vi "reference_cluster.vi"(0 "control cluster":T5, 3 "error in":errorcluster) -> (4 "error event refnum":refnum<event-registration>, 5 "reference cluster":T6, 8 "error out":errorcluster)   [LabVIEW 2016]
uses:
  Type Definitions/reference_cluster.ctl
  Type Definitions/vars_settings.ctl
  Type Definitions/stim_type.ctl
  Type Definitions/backlight_type.ctl
  Type Definitions/vars_runtime.ctl
  Type Definitions/data.ctl
  Type Definitions/notifier_elements_GUI.ctl
  Type Definitions/notifier_elements_DAQ.ctl
  Type Definitions/notifier_elements_write.ctl
  Type Definitions/control_references.ctl
panel:
  in  "vars runtime":T1[](array[typedef])=[{"t wait"=5000, "t stim"=0, "t square"=0, "t digStimOne"=0, "t digStimTwo"=0, "t rew"=0, "t onset"=0, "n stim"=0, "n hit"=0, "n miss"=0, "n catch"=0, "n reject"=0, "n false alarm"=0, "stim amp"=0.0, "stim idx"=0, "next temp"=0.0, "catch"=FALSE, "stimulus"=FALSE, "reward given"=FALSE, "penalty given"=FALSE, "lick"=FALSE, "next reward"=FALSE, "penalty"=FALSE, "backlight"=FALSE, "square"=FALSE, "digStimOne"=FALSE, "digStimTwo"=FALSE, "first run?"=FALSE, "timeout"=FALSE, "free reward"=FALSE, "pairing"=FALSE, "d stim"=0, "d square"=0, "n rew"=0, "d timeout catch"=0, "t penalty"=0}, {"t wait"=5000, "t stim"=0, "t square"=0, "t digStimOne"=0, "t digStimTwo"=0, "t rew"=0, "t onset"=0, "n stim"=0, "n hit"=0, "n miss"=0, "n catch"=0, "n reject"=0, "n false alarm"=0, "stim amp"=0.0, "stim idx"=0, "next temp"=0.0, "catch"=FALSE, "stimulus"=FALSE, "reward given"=FALSE, "penalty given"=FALSE, "lick"=FALSE, "next reward"=FALSE, "penalty"=FALSE, "backlight"=FALSE, "square"=FALSE, "digStimOne"=FALSE, "digStimTwo"=FALSE, "first run?"=FALSE, "timeout"=FALSE, "free reward"=FALSE, "pairing"=FALSE, "d stim"=0, "d square"=0, "n rew"=0, "d timeout catch"=0, "t penalty"=0}, {"t wait"=5000, "t stim"=0, "t square"=0, "t digStimOne"=0, "t digStimTwo"=0, "t rew"=0, "t onset"=0, "n stim"=0, "n hit"=0, "n miss"=0, "n catch"=0, "n reject"=0, "n false alarm"=0, "stim amp"=0.0, "stim idx"=0, "next temp"=0.0, "catch"=FALSE, "stimulus"=FALSE, "reward given"=FALSE, "penalty given"=FALSE, "lick"=FALSE, "next reward"=FALSE, "penalty"=FALSE, "backlight"=FALSE, "square"=FALSE, "digStimOne"=FALSE, "digStimTwo"=FALSE, "first run?"=FALSE, "timeout"=FALSE, "free reward"=FALSE, "pairing"=FALSE, "d stim"=0, "d square"=0, "n rew"=0, "d timeout catch"=0, "t penalty"=0}, {"t wait"=5000, "t stim"=0, "t square"=0, "t digStimOne"=0, "t digStimTwo"=0, "t rew"=0, "t onset"=0, "n stim"=0, "n hit"=0, "n miss"=0, "n catch"=0, "n reject"=0, "n false alarm"=0, "stim amp"=0.0, "stim idx"=0, "next temp"=0.0, "catch"=FALSE, "stimulus"=FALSE, "reward given"=FALSE, "penalty given"=FALSE, "lick"=FALSE, "next reward"=FALSE, "penalty"=FALSE, "backlight"=FALSE, "square"=FALSE, "digStimOne"=FALSE, "digStimTwo"=FALSE, "first run?"=FALSE, "timeout"=FALSE, "free reward"=FALSE, "pairing"=FALSE, "d stim"=0, "d square"=0, "n rew"=0, "d timeout catch"=0, "t penalty"=0}]
  in  "vars general":T2[](array[typedef])=[{"base directory"=path "", "data directory"=path "", "active"=FALSE, "running"=FALSE, "pairing"=FALSE, "clean tubes"=FALSE, "animal ID"=1, "session ID"=0, "base temp"=32.0, "d wait min"=500, "d wait max"=1000, "d timeout"=5000, "d timeout catch"=0, "d penalty"=0, "d reward"=100, "n reward"=1, "idx stim"=0, "timeout win"=5000, "lick win"=[0, 100], "stim type"=[enum."pulse", enum."sine", enum."square"], "stim dur"=[500, 700, 600], "stim amp"=[10.0, 10.0, 10.0], "stim freq"=[50, 50, 50], "stim ramp"=[50, 1, 1], "stim catch"=[0, 0, 1], "pairing delay"=[0, 0, 0], "square dur"=[50, 20, 10], "square delay"=[50, 20, 10], "square freq"=[50, 50, 50], "square dc"=[50, 20, 10], "stim shape"=[], "square shape"=[], "backlight type"=enum."random", "backlight freq"=10, "dStimOne dur"=[100, 100, 100], "dStimOne delay"=[100, 100, 100], "dStimTwo dur"=[100, 100, 100], "dStimTwo delay"=[100, 100, 100]}, {"base directory"=path "", "data directory"=path "", "active"=FALSE, "running"=FALSE, "pairing"=FALSE, "clean tubes"=FALSE, "animal ID"=2, "session ID"=0, "base temp"=32.0, "d wait min"=500, "d wait max"=1000, "d timeout"=5000, "d timeout catch"=0, "d penalty"=0, "d reward"=100, "n reward"=1, "idx stim"=0, "timeout win"=5000, "lick win"=[0, 100], "stim type"=[enum."pulse", enum."sine", enum."square"], "stim dur"=[500, 700, 600], "stim amp"=[10.0, 10.0, 10.0], "stim freq"=[50, 50, 50], "stim ramp"=[50, 1, 1], "stim catch"=[0, 0, 1], "pairing delay"=[0, 0, 0], "square dur"=[50, 20, 10], "square delay"=[50, 20, 10], "square freq"=[50, 50, 50], "square dc"=[50, 20, 10], "stim shape"=[], "square shape"=[], "backlight type"=enum."random", "backlight freq"=10, "dStimOne dur"=[100, 100, 100], "dStimOne delay"=[100, 100, 100], "dStimTwo dur"=[100, 100, 100], "dStimTwo delay"=[100, 100, 100]}, {"base directory"=path "", "data directory"=path "", "active"=FALSE, "running"=FALSE, "pairing"=FALSE, "clean tubes"=FALSE, "animal ID"=3, "session ID"=0, "base temp"=32.0, "d wait min"=500, "d wait max"=1000, "d timeout"=5000, "d timeout catch"=0, "d penalty"=0, "d reward"=100, "n reward"=1, "idx stim"=0, "timeout win"=5000, "lick win"=[0, 100], "stim type"=[enum."pulse", enum."sine", enum."square"], "stim dur"=[500, 700, 600], "stim amp"=[10.0, 10.0, 10.0], "stim freq"=[50, 50, 50], "stim ramp"=[50, 1, 1], "stim catch"=[0, 0, 1], "pairing delay"=[0, 0, 0], "square dur"=[50, 20, 10], "square delay"=[50, 20, 10], "square freq"=[50, 50, 50], "square dc"=[50, 20, 10], "stim shape"=[], "square shape"=[], "backlight type"=enum."random", "backlight freq"=10, "dStimOne dur"=[100, 100, 100], "dStimOne delay"=[100, 100, 100], "dStimTwo dur"=[100, 100, 100], "dStimTwo delay"=[100, 100, 100]}, {"base directory"=path "", "data directory"=path "", "active"=FALSE, "running"=FALSE, "pairing"=FALSE, "clean tubes"=FALSE, "animal ID"=4, "session ID"=0, "base temp"=32.0, "d wait min"=500, "d wait max"=1000, "d timeout"=5000, "d timeout catch"=0, "d penalty"=0, "d reward"=100, "n reward"=1, "idx stim"=0, "timeout win"=5000, "lick win"=[0, 100], "stim type"=[enum."pulse", enum."sine", enum."square"], "stim dur"=[500, 700, 595], "stim amp"=[10.0, 10.0, 10.0], "stim freq"=[50, 50, 50], "stim ramp"=[50, 1, 1], "stim catch"=[0, 0, 1], "pairing delay"=[0, 0, 0], "square dur"=[50, 20, 10], "square delay"=[50, 20, 10], "square freq"=[50, 50, 50], "square dc"=[50, 20, 10], "stim shape"=[], "square shape"=[], "backlight type"=enum."random", "backlight freq"=10, "dStimOne dur"=[100, 100, 100], "dStimOne delay"=[100, 100, 100], "dStimTwo dur"=[100, 100, 100], "dStimTwo delay"=[100, 100, 100]}] {"stim ramp" min=1}
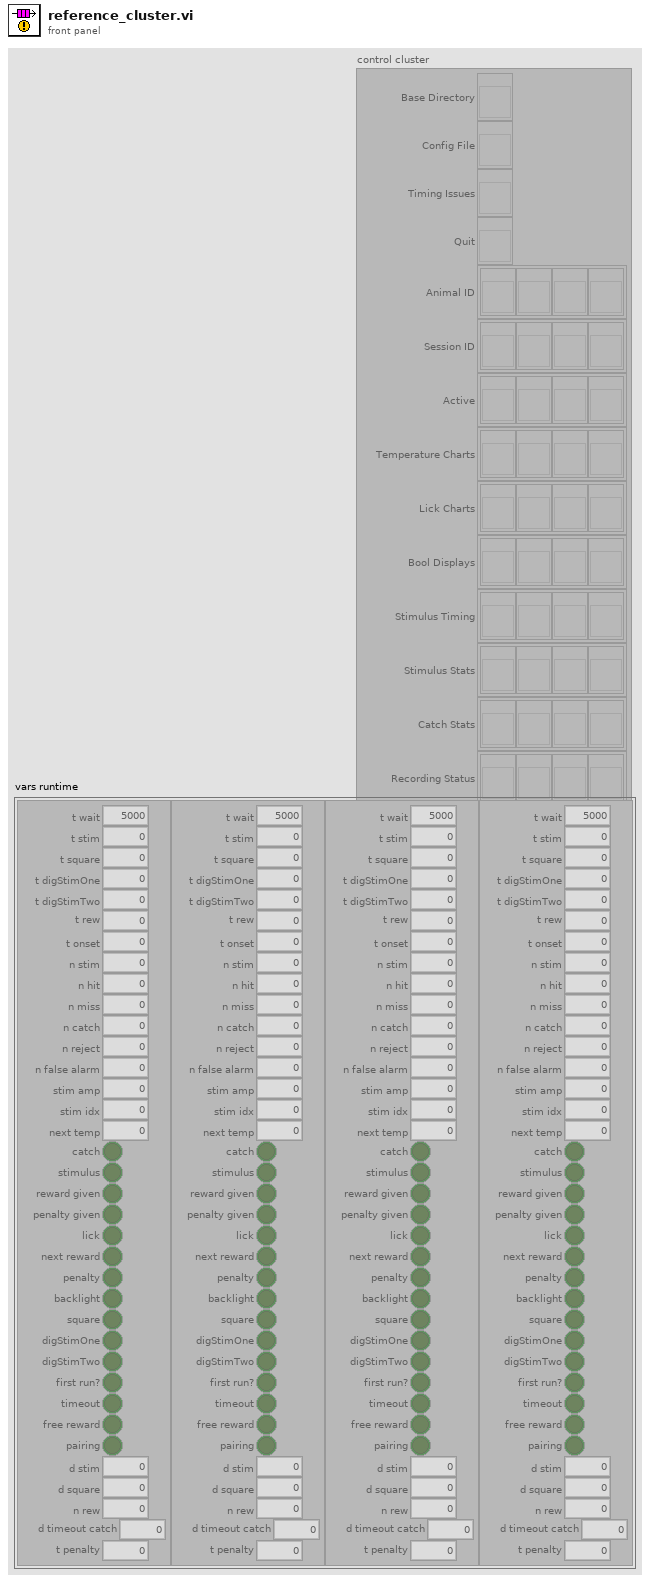
[diagram p1: front panel]
types:
  T1 = typedef "vars_runtime.ctl" = cluster{"t wait":u16, "t stim":u16, "t square":u16, "t digStimOne":u16, "t digStimTwo":u16, "t rew":u16, "t onset":u32, "n stim":u16, "n hit":u16, "n miss":u16, "n catch":u16, "n reject":u16, "n false alarm":u16, "stim amp":sgl, "stim idx":i32, "next temp":sgl, "catch":bool, "stimulus":bool, "reward given":bool, "penalty given":bool, "lick":bool, "next reward":bool, "penalty":bool, "backlight":bool, "square":bool, "digStimOne":bool, "digStimTwo":bool, "first run?":bool, "timeout":bool, "free reward":bool, "pairing":bool, "d stim":u16, "d square":u16, "n rew":u16, "d timeout catch":u16, "t penalty":u16}
  T2 = typedef "vars_settings.ctl" = cluster{"base directory":path, "data directory":path, "active":bool, "running":bool, "pairing":bool, "clean tubes":bool, "animal ID":u16, "session ID":u16, "base temp":dbl, "d wait min":u16, "d wait max":u16, "d timeout":u16, "d timeout catch":u16, "d penalty":u16, "d reward":u16, "n reward":u16, "idx stim":u16, "timeout win":u16, "lick win":i32[], "stim type":T3[], "stim dur":u16[], "stim amp":dbl[], "stim freq":u16[], "stim ramp":u16[], "stim catch":u8[], "pairing delay":i16[], "square dur":u16[], "square delay":i16[], "square freq":u8[], "square dc":u8[], "stim shape":dbl[][], "square shape":bool[][], "backlight type":T4, "backlight freq":u16, "dStimOne dur":u16[], "dStimOne delay":i16[], "dStimTwo dur":u16[], "dStimTwo delay":i16[]}
  T3 = typedef "stim_type.ctl" = enum16{"pulse", "vibration", "square", "sine"}
  T4 = typedef "backlight_type.ctl" = enum16{"none", "random", "regular"}
  T5 = typedef "control_references.ctl" = cluster{"Base Directory":refnum<vi>, "Config File":refnum<vi>, "Timing Issues":refnum<vi>, "Quit":refnum<vi>, "Animal ID":refnum<vi>[], "Session ID":refnum<vi>[], "Active":refnum<vi>[], "Temperature Charts":refnum<vi>[], "Lick Charts":refnum<vi>[], "Bool Displays":refnum<vi>[], "Stimulus Timing":refnum<vi>[], "Stimulus Stats":refnum<vi>[], "Catch Stats":refnum<vi>[], "Recording Status":refnum<vi>[], "Pairing":refnum<vi>[]}
  T6 = typedef "reference_cluster.ctl" = cluster{"Vars":cluster{"General":refnum<notifier>, "Runtime":refnum<notifier>}, "Data":cluster{"Display":refnum<queue>, "Write":refnum<queue>}, "LoopCtrl":cluster{"Display":refnum<notifier>, "DAQ":refnum<notifier>, "Write":refnum<notifier>[]}, "Controls":T5, "Error Event":refnum<user-event>}
  T7 = typedef "data.ctl" = cluster{"time":dbl, "finished late":bool, "temp out":sgl[], "temp in":sgl[], "lick in":sgl[], "stim":bool[], "catch":bool[], "lick":bool[], "reward":bool[], "penalty":bool[], "backlight":bool[], "freqstim":bool[], "dStimOne":bool[], "dStimTwo":bool[], "free reward":bool[], "timeout":bool[], "pairing":bool[]}
  T8 = typedef "notifier_elements_write.ctl" = enum16{"Initialize", "Pause", "Write Data", "Close Files", "Quit"}
  T9 = typedef "notifier_elements_GUI.ctl" = enum16{"Initialize GUI", "Pause", "Live Update", "Stat Update", "Quit"}
  T10 = typedef "notifier_elements_DAQ.ctl" = enum16{"DAQ - Initialize", "DAQ - Pause", "DAQ - Run", "DAQ - Quit"}
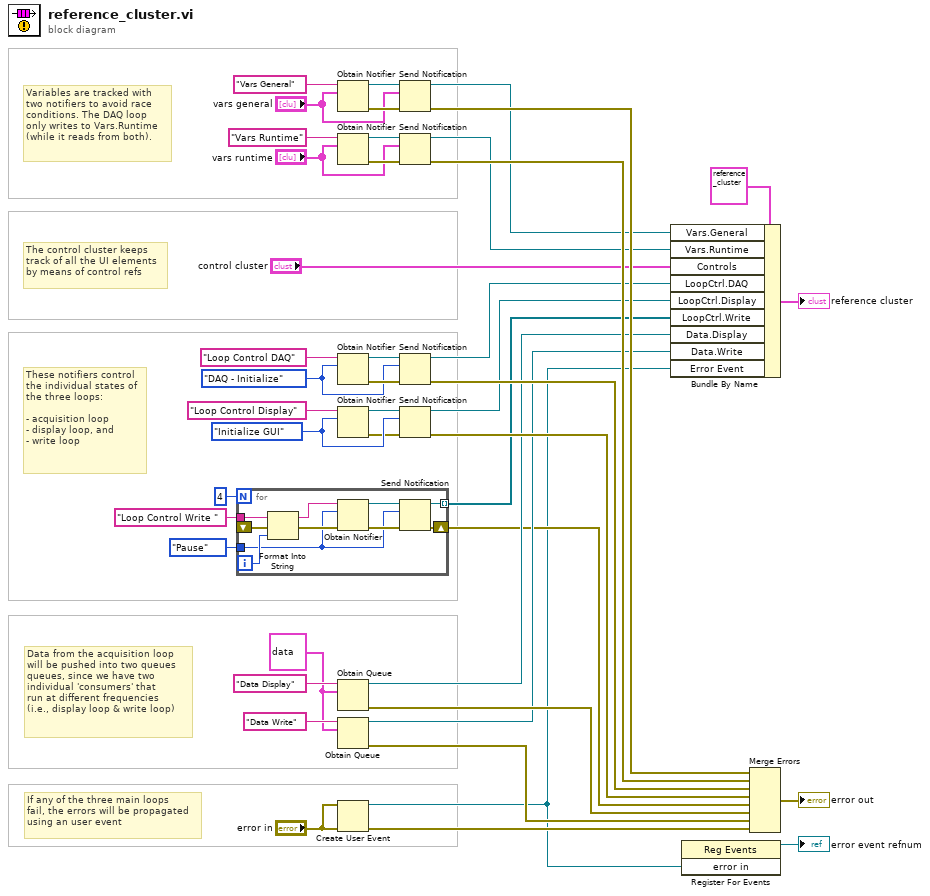
[diagram p0: block diagram]
diagram:
  w26 = T7 {"time"=0.0, "finished late"=FALSE, "temp out"=[], "temp in"=[], "lick in"=[], "stim"=[], "catch"=[], "lick"=[], "reward"=[], "penalty"=[], "backlight"=[], "freqstim"=[], "dStimOne"=[], "dStimTwo"=[], "free reward"=[], "timeout"=[], "pairing"=[]} ("Data")
  w35 = notifier_elements_GUI."Initialize GUI" ("GUI init")
  w36 = notifier_elements_DAQ."DAQ - Initialize" ("DAQ init")
  # "If any of the three main loops\nfail, the errors will be propagated\nusing an user event"
  # "Variables are tracked with\ntwo notifiers to avoid race\nconditions. The DAQ loop\nonly writes to Vars.Runtime\n(while it reads from both)."
  # "The control cluster keeps\ntrack of all the UI elements\nby means of control refs"
  # "Data from the acquisition loop\nwill be pushed into two queues\nqueues, since we have two\nindividual 'consumers' that\nrun at different frequencies\n(i.e., display loop & write loop)"
  # "These notifiers control\nthe individual states of\nthe three loops:\n\n- acquisition loop\n- display loop, and\n- write loop"
  n1 = for {
    N: 4 -> [_]
    tunnel: notifier_elements_write."Pause" ("Write init") -> [w45]
    shift-right: [w47] -> w11
    shift-left: _ -> [w54]
    tunnel: [w46] -> w9 mode=indexing
    tunnel: "Loop Control Write " ("name (unnamed)") -> [w53]
    i -> [w50]
    n2 = Format Into String(initial string=w53, error in=w54, w50) -> (resulting string=w51:string, error out=w52:errorcluster)  [unwired: 1 in]
    n3 = Obtain Notifier(name (unnamed)=w51, notification data type=w45, error in (no error)=w52) -> (notifier out=w49:refnum<notifier>, error out=w48:errorcluster)  [unwired: 1 in, 1 out]
    n4 = Send Notification(notification=w45, notifier=w49, error in (no error)=w48) -> (notifier out=w46:refnum<notifier>, error out=w47:errorcluster)
  }
  n5 = Obtain Notifier(name (unnamed)="Vars General", notification data type="vars general") -> (notifier out=w22:refnum<notifier>, error out=w21:errorcluster)  [unwired: 2 in, 1 out]
  n6 = Obtain Notifier(name (unnamed)="Vars Runtime", notification data type="vars runtime") -> (notifier out=w18:refnum<notifier>, error out=w19:errorcluster)  [unwired: 2 in, 1 out]
  n7 = Obtain Notifier(name (unnamed)="Loop Control DAQ", notification data type=w36) -> (notifier out=w38:refnum<notifier>, error out=w39:errorcluster)  [unwired: 2 in, 1 out]
  n8 = Obtain Notifier(name (unnamed)="Loop Control Display", notification data type=w35) -> (notifier out=w33:refnum<notifier>, error out=w32:errorcluster)  [unwired: 2 in, 1 out]
  n9 = Obtain Queue(name (unnamed)="Data Display", element data type=w26) -> (queue out=w23:refnum<queue>, error out=w40:errorcluster)  [unwired: 3 in, 1 out]
  n10 = Obtain Queue(name (unnamed)="Data Write", element data type=w26) -> (queue out=w24:refnum<queue>, error out=w25:errorcluster)  [unwired: 3 in, 1 out]
  n11 = Create User Event(user event datatype="error in", error in="error in") -> (user event=w2:refnum<user-event>, error out=w3:errorcluster)
  n12 = Send Notification(notification="vars general", notifier=w22, error in (no error)=w21) -> (notifier out=w15:refnum<notifier>, error out=w41:errorcluster)
  n13 = Send Notification(notification="vars runtime", notifier=w18, error in (no error)=w19) -> (notifier out=w16:refnum<notifier>, error out=w42:errorcluster)
  n14 = Send Notification(notification=w36, notifier=w38, error in (no error)=w39) -> (notifier out=w31:refnum<notifier>, error out=w43:errorcluster)
  n15 = Send Notification(notification=w35, notifier=w33, error in (no error)=w32) -> (notifier out=w30:refnum<notifier>, error out=w44:errorcluster)
  n16 = Bundle By Name(cluster=T6 {"Vars"={"General"=refnum, "Runtime"=refnum}, "Data"={"Display"=refnum, "Write"=refnum}, "LoopCtrl"={"Display"=refnum, "DAQ"=refnum, "Write"=[]}, "Controls"={"Base Directory"=refnum, "Config File"=refnum, "Timing Issues"=refnum, "Quit"=refnum, "Animal ID"=[], "Session ID"=[], "Active"=[], "Temperature Charts"=[], "Lick Charts"=[], "Bool Displays"=[], "Stimulus Timing"=[], "Stimulus Stats"=[], "Catch Stats"=[], "Recording Status"=[], "Pairing"=[]}, "Error Event"=refnum} ("notifier cluster"), "Vars.General"=w15, "Vars.Runtime"=w16, "Controls"="control cluster", "LoopCtrl.DAQ"=w31, "LoopCtrl.Display"=w30, "LoopCtrl.Write"=w9, "Data.Display"=w23, "Data.Write"=w24, "Error Event"=w2) -> (→"reference cluster":T6)
  n17 = register-events(w2) -> (reference out=→"error event refnum":refnum<event-registration>)  [unwired: 2 in, 1 out]
  n18 = Merge Errors(w41, w42, w43, w44, w11, w40, w25, w3) -> (→"error out":errorcluster)
